vi "Destroy All Channels.vi"(8 "error in (no error)":errorcluster, 11 "CIFChannelMng in":refnum<class "CIFChannelMng.lvclass">) -> (0 "error out":errorcluster, 3 "CIFChannelMng out":refnum<class "CIFChannelMng.lvclass">)   [LabVIEW 2021, in "CIFChannelMng.lvclass"]
uses:
  CIFChannelMng.lvclass
  CIFChannelMng.lvclass/CIFChannelMng.ctl
  CIFChannels/CIFChannels.lvclass
  CIFChannels/Typedef/Direction.ctl
  typedef/Channel List for OOB.ctl
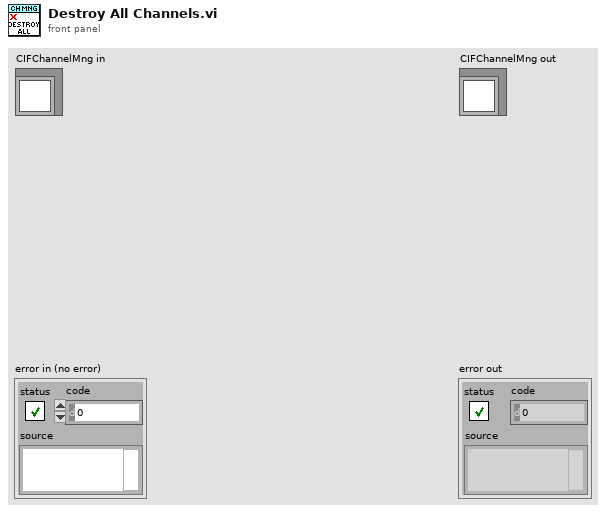
[diagram p1: front panel]
types:
  T1 = typedef "CIFChannelMng.lvclass/Channel List for OOB.ctl" = cluster{"Direction":T2, "Type":string, "Connected?":bool, "Connected Name":string, "Custom Config Data":u8[]}
  T2 = typedef "CIFChannels.lvclass/Direction.ctl" = enum16{"Publisher", "Subscriber"}
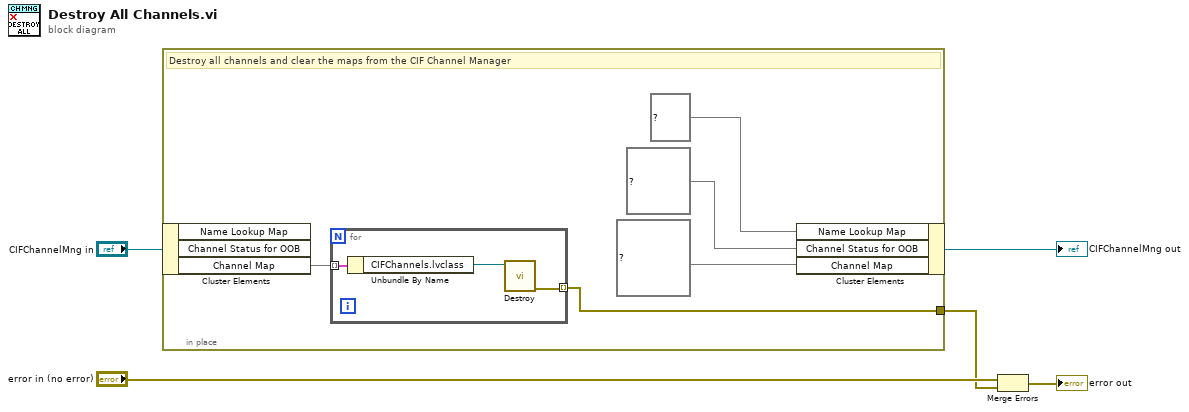
[diagram p0: block diagram]
diagram:
  n1 = in-place {
    in-place-border: [w7] -> w2
    # "Destroy all channels and clear the maps from the CIF Channel Manager"
    n2 = in-place-cluster #1("CIFChannelMng in") -> ("Channel Map"=w10:map{string, refnum<class "CIFChannels.lvclass">})  [unwired: 2 out]
    n3 = for {
      tunnel: w10 -> [w13] mode=indexing
      tunnel: [w11] -> w7 mode=indexing
      n4 = Unbundle By Name(w13) -> ("CIFChannels.lvclass"=w12:refnum<class "CIFChannels.lvclass">)
      n5 = call-dynamic "Destroy.vi"("CIFChannels in"=w12) -> ("error out"=w11:errorcluster)  [unwired: 9 in, 1 out]
    }
    n6 = in-place-cluster #1("Name Lookup Map"=map{u16, string} {}, "Channel Status for OOB"=map{string, T1} {}, "Channel Map"=map{string, refnum<class "CIFChannels.lvclass">} {}) -> (→"CIFChannelMng out":refnum<class "CIFChannelMng.lvclass">)
  }
  n7 = Merge Errors("error in (no error)", w2) -> (→"error out":errorcluster)
